vi "Select Plot.vi"(0 "State":T1) -> ()   [LabVIEW 2020, in "Interactive Graph.xctl"]
uses:
  Interactive Graph.xctl
  State.vi
  Persistent.ctl
  Plot.ctl
  EPhys/LV Source/Work Panel VIs/Typedefs/EPhysWork-Label Position.ctl
  Events.ctl
  Selection.ctl
  XRange.ctl
  YScale.ctl
  Cursor.ctl
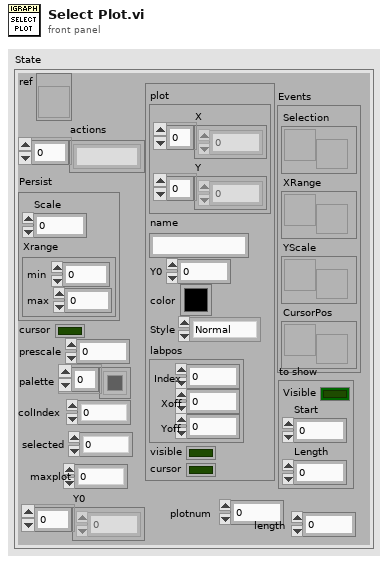
[diagram p1: front panel]
types:
  T1 = typedef "Interactive Graph.xctl/State.vi" = cluster{"ref":refnum<vi>, "actions":string[], "Persist":T2, "cursor":bool, "prescale":dbl, "palette":u32[], "colIndex":i32, "to add":T3, "Events":T5, "selected":i32, "to show":cluster{"Visible":bool, "Start":i32, "Length":i32}, "maxplot":i32, "Y0":dbl[], "plotnum":i32, "length":i32}
  T2 = typedef "Interactive Graph.xctl/Persistent.ctl" = cluster{"Scale":dbl, "Xrange":cluster{"min":dbl, "max":dbl}}
  T3 = typedef "Interactive Graph.xctl/Plot.ctl" = cluster{"plot":cluster{"X":dbl[], "Y":dbl[]}, "name":string, "Y0":dbl, "color":u32, "Style":enum16{"Normal", "Highlight", "Shadow"}, "labpos":T4, "visible":bool, "cursor":bool}
  T4 = typedef "EPhysWork-Label Position.ctl" = cluster{"Index":i32, "Xoff":dbl, "Yoff":dbl}
  T5 = typedef "Interactive Graph.xctl/Events.ctl" = cluster{"Selection":refnum<user-event>, "XRange":refnum<user-event>, "YScale":refnum<user-event>, "CursorPos":refnum<user-event>}
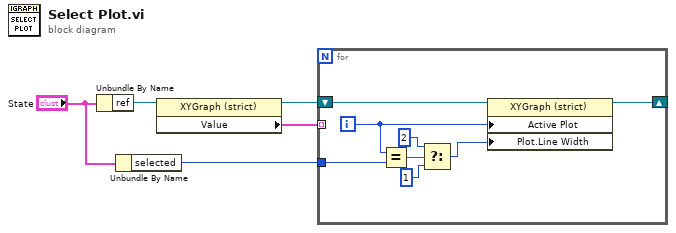
[diagram p0: block diagram]
diagram:
  n1 = Unbundle By Name("State") -> ("ref"=w5:refnum<vi>)
  n2 = Unbundle By Name("State") -> ("selected"=w1:i32)
  n3 = property class="XYGraph (strict)"(reference=w5) -> (reference out=w3:refnum<vi>, "Value"=w4:cluster{dbl[], dbl[]}[])  [unwired: 1 in, 1 out]
  n4 = for {
    tunnel: w4 -> [_] mode=indexing
    shift-right: [w10] -> _
    shift-left: w3 -> [w13]
    tunnel: w1 -> [w11]
    i -> [w12]
    n5 = Equal?(x=w12, y=w11) -> (x = y?=w9:bool)
    n6 = Select(t=2, s=w9, f=1) -> (s? t:f=w7:i32)
    n7 = property class="XYGraph (strict)"(reference=w13, "Active Plot"=w12, "Plot.Line Width"=w7) -> (reference out=w10:refnum<vi>)  [unwired: 1 in, 1 out]
  }
